vi "16 - Fonts (Render As Surface).vi"() -> ()   [LabVIEW 2015]
uses:
  Libraries/LibSDL2 Wrapper/Controls/Init Flags.ctl
  Libraries/LibSDL2 Wrapper/Controls/NULL.ctl
  Libraries/LibSDL2 Wrapper/LibSDL2.lvlib
  Libraries/LibSDL2_Image Wrapper/LibSDL2_Image.lvlib
  Libraries/LibSDL2_TTF Wrapper/LibSDL2_TTF.lvlib
panel:
  in  "Colour":u32(colorbox)=16448250
  in  "stop":bool
  out "Error":string
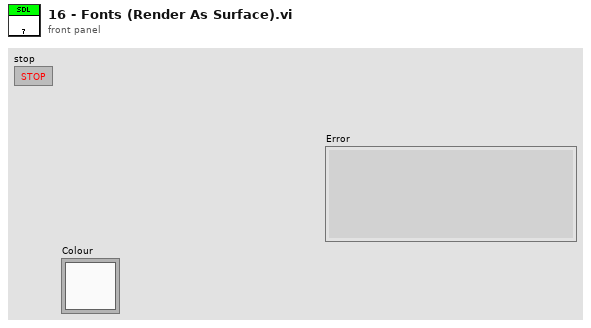
[diagram p1: front panel]
types:
  T1 = typedef "LibSDL2.lvlib/Init Flags.ctl" = u32
  T2 = typedef "LibSDL2.lvlib/NULL.ctl" = enum32{"NULL"}
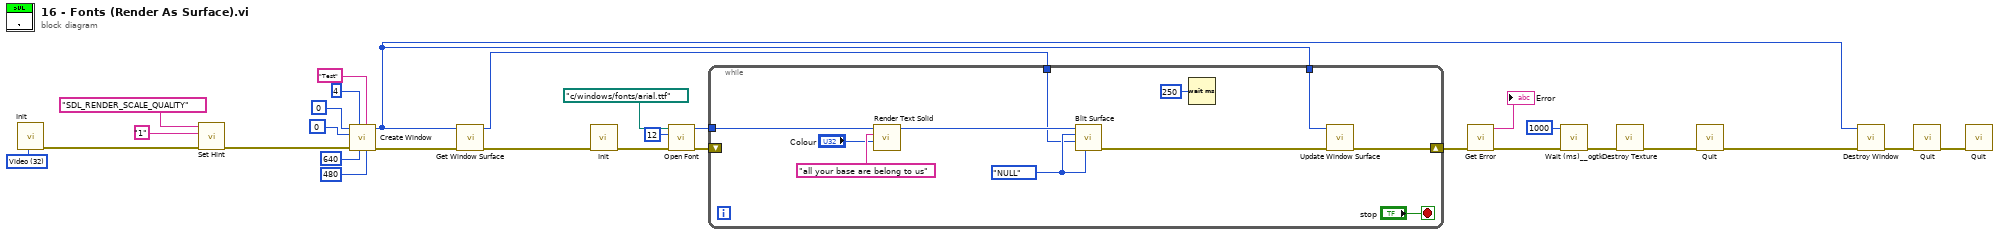
[diagram p0: block diagram]
diagram:
  w29 = T1 32 items=["Timer"=1, "Audio"=16, "Video"=32, "Joystick"=512, "Haptic"=4096, "Game Controller"=8192, "Events"=16384, "No Parachute"=1048576, "Everything"=17244689] ("Init Flags")
  n1 = call "Init.vi"("Flags"=w29) -> ("error out"=w20:errorcluster)  [unwired: 9 in, 1 out]
  n2 = call "Set Hint.vi"("error in"=w20, "Value"="1", "Name"="SDL_RENDER_SCALE_QUALITY") -> ("error out"=w19:errorcluster)  [unwired: 7 in, 1 out]
  n3 = call "Create Window.vi"("Height"=480, "Title"="Test", "Width"=640, "Flags"=u32 4, "error in"=w19, "Position y"=u32 0 ("Flags"), "Position x"=u32 0 ("Flags")) -> ("error out"=w6:errorcluster, "Window Pointer"=w4:u32)  [unwired: 3 in]
  n4 = call "Get Window Surface.vi"("error in"=w6, "Window Pointer"=w4) -> ("error out"=w5:errorcluster, "Surface Pointer"=w2:u32)  [unwired: 8 in]
  n5 = call "Init.vi"("error in (no error)"=w5) -> ("error out"=w11:errorcluster)  [unwired: 9 in, 1 out]
  n6 = call "Open Font.vi"("error in (no error)"=w11, "Size"=12, "File"=path "c:/windows/fonts/arial.ttf") -> ("error out"=w10:errorcluster, "Font Pointer"=w9:u32)  [unwired: 7 in]
  n7 = while {
    tunnel: w9 -> [w40]
    tunnel: w4 -> [w37]
    tunnel: w2 -> [w32]
    shift-right: [w35] -> w3
    shift-left: w10 -> [_]
    stop <- "stop" stop-if-true
    w34 = NULL."NULL" ("Null")
    n8 = call "Render Text Solid.vi"("Colour"="Colour", "Text"="all your base are belong to us", "Font Pointer"=w40) -> ("Surface Pointer"=w38:u32)  [unwired: 8 in]
    n9 = call "Blit Surface.vi"("Destination Rectangle Pointer"=w34, "Destination Surface Pointer"=w32, "Source Rectangle Pointer"=w34, "Source Surface Pointer"=w38) -> ("error out"=w36:errorcluster)  [unwired: 6 in, 1 out]
    n10 = Wait (ms)(milliseconds to wait=u32 250) -> ()  [unwired: 1 out]
    n11 = call "Update Window Surface.vi"("error in"=w36, "Window Pointer"=w37) -> ("error out"=w35:errorcluster)  [unwired: 9 in]
  }
  n12 = call "Get Error.vi"("error in"=w3) -> ("error out"=w12:errorcluster, "Error"=→"Error":string)  [unwired: 9 in]
  n13 = call <userlib>:"Wait (ms)__ogtk.vi"("error in (no error)"=w12, "milliseconds to wait"=u32 1000) -> ("error out"=w13:errorcluster)  [unwired: 8 in, 1 out]
  n14 = call "Destroy Texture.vi"("error in"=w13) -> ("error out"=w16:errorcluster)  [unwired: 10 in]
  n15 = call "Quit.vi"("error in (no error)"=w16) -> ("error out"=w1:errorcluster)  [unwired: 10 in]
  n16 = call "Destroy Window.vi"("error in"=w1, "Window Pointer"=w4) -> ("error out"=w22:errorcluster)  [unwired: 9 in]
  n17 = call "Quit.vi"("error in"=w22) -> ("error out"=w21:errorcluster)  [unwired: 10 in]
  n18 = call "Quit.vi"("error in"=w21) -> ()  [unwired: 10 in, 1 out]
